vi "子VI-查看某框-只读穿透图模式.vi"(0 "输入框号（默认值0为整张图）":dbl format="%#_13g", 1 "框组":T3(array[cluster]), 3 "临界Z值":i32, 4 "弥散类缺陷灰度阈值":dbl caption="值", 5 "临界面积百分比值":dbl, 6 "分层缺陷的面积阈值":i32, 7 "预先配置的灰度阈值":dbl, 8 "穿透图原始路径":path, 9 "部位信息":string[](array[string])=["", "34.500000", "32.500000", "1121", "34", "54.955926", "分层类", "不合格", ""], 16 "产品规格":cluster{"产品长度（周长）（mm）":dbl, "产品宽度（母线长）（mm）":dbl}) -> (27 "全部检测结果":string[][](table))   [LabVIEW 2018]
uses:
  <vilib>/vision/NI_Vision_Development_Module.lvlib
panel:
  out "分层类缺陷低于阈值的累计面积":dbl
  out "中心Y":dbl
  out "中心X":dbl
  in  "格式字符串 4":string="%f"
  in  "分隔符（'\\'代码显示） 3":string="\t"
  out "?":string[][](table)
  in  "返回主界面":bool caption="辅助定性分析"
  in  "Tab Control":T1
  out "?":T2(plugin-control)
  out "Threshold Image":T2(plugin-control)
  out "Threshold Image":T2(plugin-control)
  in  "格式字符串 3":string="%f"
  in  "分隔符（'\\'代码显示） 2":string="\t"
  out "弥散缺陷个数":i32
  out "分层缺陷个数":i32
  out "合格？ 弥散类":string="fencengThreshold"
  out "合格？分层类":string="fencengThreshold"
  out "弥散测量结果":dbl[][](array[numeric])
  out "弥散类检测结果":string[][](table)
  out "?":string
  out "面积 (pixels)":i32
  in  "格式字符串 2":string="%f"
  in  "分隔符（'\\'代码显示）":string="\t"
  out "分层测量结果":dbl[][](array[numeric])
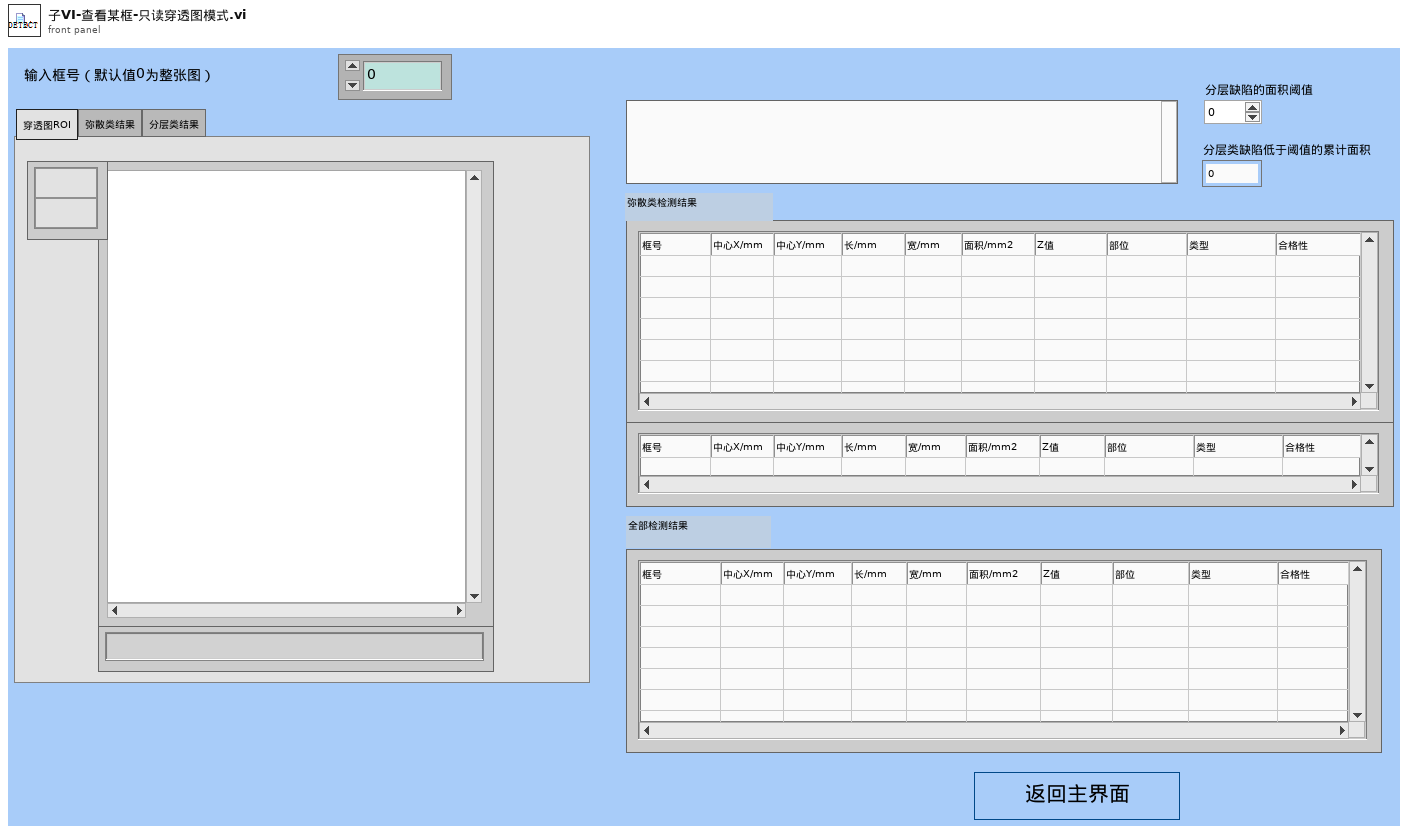
[diagram p1: front panel]
types:
  T1 = typedef "控件2.ctl" = enum32{"穿透图ROI", "弥散类结果", "分层类结果"}
  T2 = typedef "IMAQ Image.ctl" = refnum<image>
  T3 = cluster{"Global Rectangle":i32[], "Contours":cluster{"Contour Type":u32, "ROI Type":u32, "Points":i32[]}[]}[]
  T4 = cluster{"Zoom Tool":bool, "Selection Tool":bool, "Pan Tool":bool, "Point Tool":bool, "Line Tool":bool, "Rectangle Tool":bool, "Rotated Rectangle Tool":bool, "Polyline Tool":bool, "Polygon Tool":bool, "Freehand Tool":bool, "Closed Freehand Tool":bool, "Ellipse Tool":bool, "Annulus Tool":bool}
  T5 = typedef "Image Type" = u32
  T6 = cluster{"Global Rectangle":i32[], "Contours":cluster{"Contour Type":u32, "ROI Type":u32, "Points":i32[]}[]}
  T7 = cluster{"histogram":u32[], "Minimal Value":sgl, "Maximal Value":sgl, "Starting Value":sgl, "Interval Width":sgl, "Mean Value":sgl, "Standard  Variation":sgl, "Area (pixels)":i32}
  T8 = cluster{"Area":dbl, "Number of Holes":dbl, "Bounding Rect":cluster{"Left":dbl, "Top":dbl, "Right":dbl, "Bottom":dbl}, "Center of Mass":cluster{"X":dbl, "Y":dbl}, "Orientation":dbl, "Dimensions":cluster{"Width":dbl, "Height":dbl}}[]
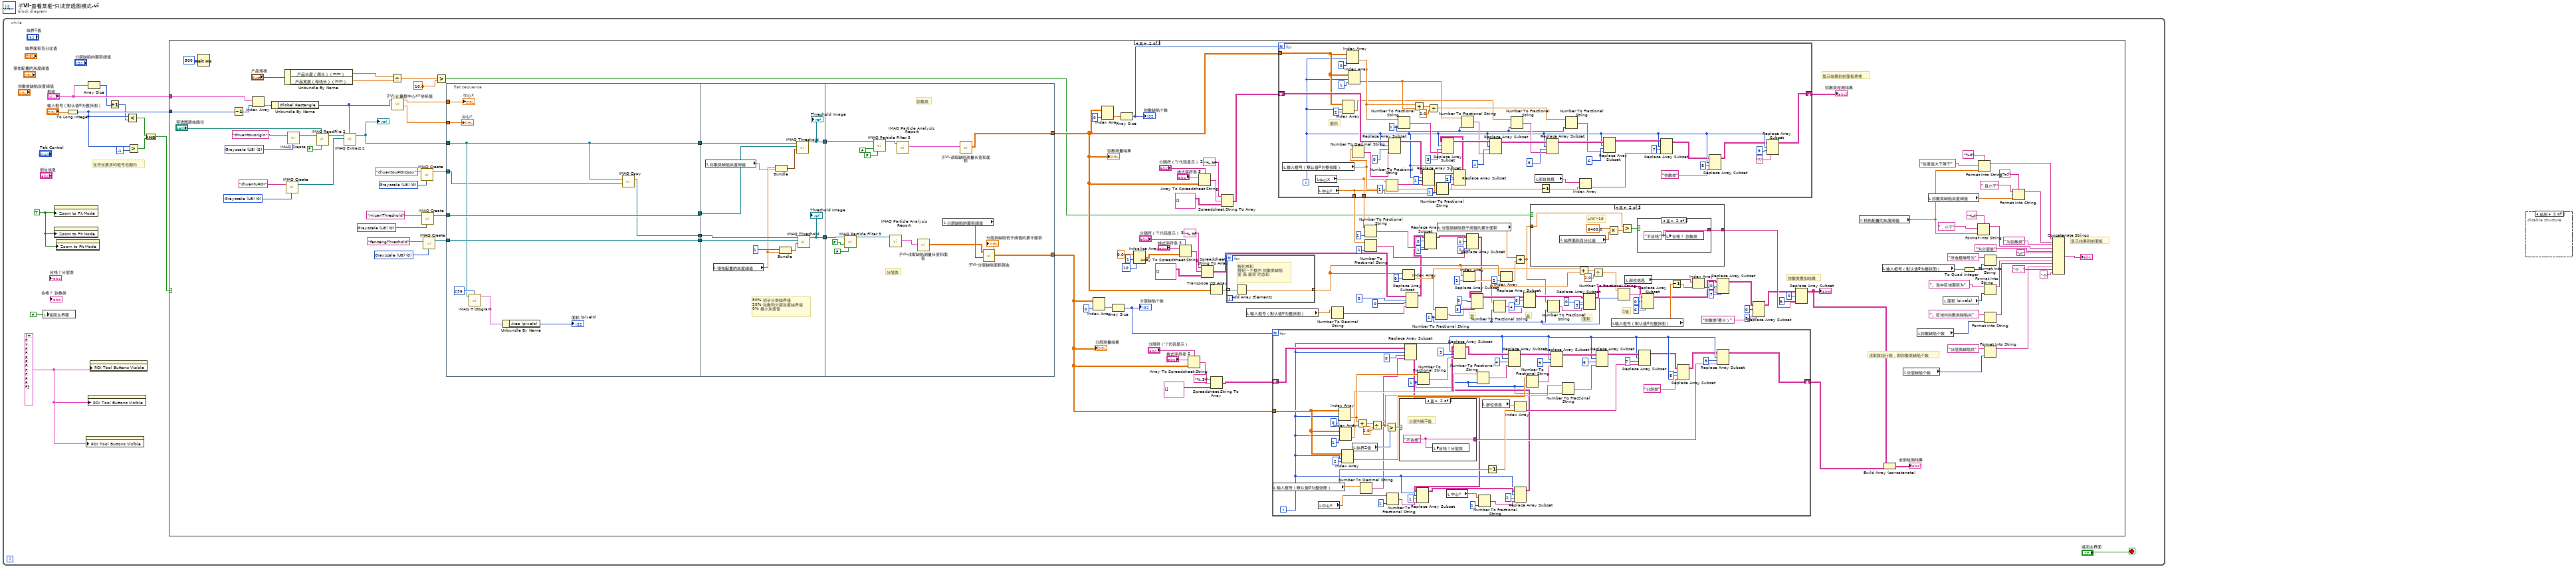
[diagram p0: block diagram]
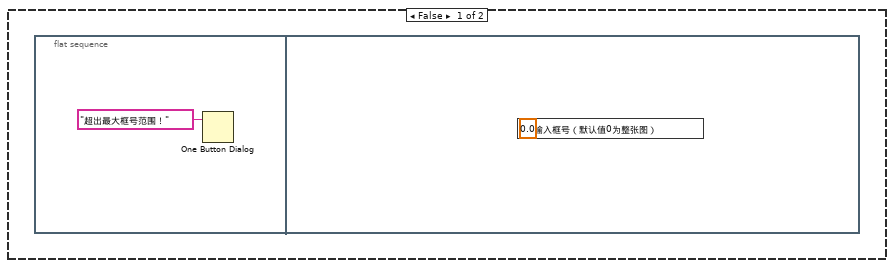
[diagram p2: hidden frame]
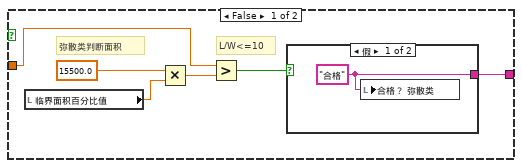
[diagram p3: hidden frame]
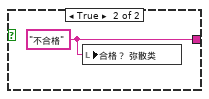
[diagram p4: hidden frame]
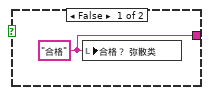
[diagram p5: hidden frame]
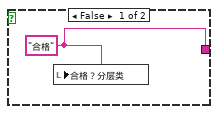
[diagram p6: hidden frame]
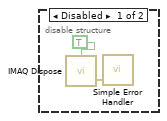
[diagram p7: hidden frame]
diagram:
  n1 = while {
    stop <- "返回主界面" stop-if-true
    w3 = T4 {"Zoom Tool"=TRUE, "Selection Tool"=FALSE, "Pan Tool"=TRUE, "Point Tool"=FALSE, "Line Tool"=FALSE, "Rectangle Tool"=FALSE, "Rotated Rectangle Tool"=FALSE, "Polyline Tool"=FALSE, "Polygon Tool"=FALSE, "Freehand Tool"=FALSE, "Closed Freehand Tool"=FALSE, "Ellipse Tool"=FALSE, "Annulus Tool"=FALSE} ("ROI Tool Buttons Visible:All Elements")
    w11 = TRUE ("Zoom to Fit Mode")
    # "在符合要求的框号范围内"
    n2 = local write "返回主界面"(FALSE ("stop")) -> ()
    n3 = property class="ImageControl"("Zoom to Fit Mode"=w11) -> ()  [unwired: 2 in, 2 out]
    n4 = property class="ImageControl"("Zoom to Fit Mode"=w11) -> ()  [unwired: 2 in, 2 out]
    n5 = property class="ImageControl"("Zoom to Fit Mode"=w11) -> ()  [unwired: 2 in, 2 out]
    n6 = To Long Integer(number="输入框号（默认值0为整张图）") -> (32bit integer=w5:i32)
    n7 = property class="ImageControl"("ROI Tool Buttons Visible"=w3) -> ()  [unwired: 2 in, 2 out]
    n8 = Array Size(array="框组") -> (size(s)=w2:i32)
    n9 = property class="ImageControl"("ROI Tool Buttons Visible"=w3) -> ()  [unwired: 2 in, 2 out]
    n10 = property class="ImageControl"("ROI Tool Buttons Visible"=w3) -> ()  [unwired: 2 in, 2 out]
    n11 = Increment(x=w2) -> (x+1=w1:i32)
    n12 = Less?(x=w5, y=w1) -> (x < y?=w7:bool)
    n13 = Greater?(x=w5, y=-1) -> (0:w6:bool)
    n14 = And(x=w7, y=w6) -> (x .and. y?=w8:bool)
    n15 = case shown="真" w8 {
      tunnel: "框组" -> [_ w106]
      tunnel: w5 -> [_ w105]
      frame False {
        n16 = flat-sequence {
          frame #0 {
            n17 = One Button Dialog(message="超出最大框号范围！" ("消息")) -> ()  [unwired: 1 in, 1 out]
          }
          frame #1 {
            n18 = local write "输入框号（默认值0为整张图）"(0.0 ("框号")) -> ()
          }
        }
      }
      frame True {
        w32 = i16 1 ("精度(6)")
        w131 = T5 0 items=["Grayscale (U8)", "Grayscale (I16)", "Grayscale (SGL)", "Complex (CSG)", "RGB (U32)", "HSL (U32)", "RGB (U64)", "Grayscale (U16)"] ("Image Type")
        w153 = T5 0 items=["Grayscale (U8)", "Grayscale (I16)", "Grayscale (SGL)", "Complex (CSG)", "RGB (U32)", "HSL (U32)", "RGB (U64)", "Grayscale (U16)"] ("Image Type")
        w154 = T5 0 items=["Grayscale (U8)", "Grayscale (I16)", "Grayscale (SGL)", "Complex (CSG)", "RGB (U32)", "HSL (U32)", "RGB (U64)", "Grayscale (U16)"] ("Image Type")
        w157 = T5 0 items=["Grayscale (U8)", "Grayscale (I16)", "Grayscale (SGL)", "Complex (CSG)", "RGB (U32)", "HSL (U32)", "RGB (U64)", "Grayscale (U16)"] ("Image Type")
        w170 = T5 0 items=["Grayscale (U8)", "Grayscale (I16)", "Grayscale (SGL)", "Complex (CSG)", "RGB (U32)", "HSL (U32)", "RGB (U64)", "Grayscale (U16)"] ("Image Type")
        # "Z值"
        # "面积"
        # "高"
        # "宽"
        # "弥散类累加结果"
        # "显示结果到前面板"
        # "读取数组行数，即弥散类缺陷个数"
        # "显示结果到前面板表格"
        n19 = Wait (ms)(milliseconds to wait=u32 500 ("等待时间（毫秒）")) -> ()  [unwired: 1 out]
        n20 = Decrement(x=w105) -> (x-1=w172:i32)
        n21 = Index Array(array=w106, index=w172) -> (element=w173:T6)
        n22 = Unbundle By Name(w173) -> ("Global Rectangle"=w48:i32[])
        n23 = Unbundle By Name("产品规格") -> ("产品长度（周长）（mm）"=w164:dbl, "产品宽度（母线长）（mm）"=w163:dbl)
        n24 = call "IMAQ Create"("Image Name"="chuantuROI", "Image Type"=w157) -> ("New Image"=w156:T2)  [unwired: 3 in, 1 out]
        n25 = call "IMAQ Create"("Image Name"="chuantouorigin", "Image Type"=w170) -> ("New Image"=w159:T2)  [unwired: 3 in, 1 out]
        n26 = call "IMAQ ReadFile 2"("Use File Path Image Type"=FALSE, "File Path"="穿透图原始路径", "Image"=w159) -> ("Image Out"=w160:T2)  [unwired: 4 in, 4 out]
        n27 = call "IMAQ Extract 2"("Optional Rectangle"=w48, "Image Dst"=w156, "Image Src"=w160) -> ("Image Dst Out"=w134:T2)  [unwired: 7 in, 1 out]
        "?" <- w134
        n28 = Divide(x=w164, y=w163) -> (x/y=w167:dbl)
        n29 = call "子VI-计算框中心XY坐标值.vi"("Global Rectangle"=w48) -> ("中心Y"=w28:dbl, "中心X"=w27:dbl)  [unwired: 9 in]
        n30 = call "IMAQ Create"("Image Name"="chuantouROIcopy", "Image Type"=w131) -> ("New Image"=w133:T2)  [unwired: 3 in, 1 out]
        n31 = call "IMAQ Create"("Image Name"="misanThreshold", "Image Type"=w153) -> ("New Image"=w148:T2)  [unwired: 3 in, 1 out]
        n32 = call "IMAQ Create"("Image Name"="fencengThreshold", "Image Type"=w154) -> ("New Image"=w147:T2)  [unwired: 3 in, 1 out]
        n33 = Greater?(x=w167, y=10.0) -> (0:w58:bool)
        n34 = flat-sequence {
          tunnel: [w261] -> w179
          tunnel: [w260] -> w178
          tunnel: [w256] -> w177
          tunnel: [w255] -> w176
          tunnel: w148 -> [w261]
          tunnel: w147 -> [w260]
          tunnel: w134 -> [w256]
          tunnel: w133 -> [w254]
          tunnel: w28 -> [w253]
          tunnel: w27 -> [w252]
          tunnel: w179 -> [w272]
          tunnel: w178 -> [w271]
          tunnel: [w267] -> w175
          tunnel: [w269] -> w174
          tunnel: w177 -> [w270]
          tunnel: w176 -> [w268]
          tunnel: [w277] -> w101
          tunnel: w175 -> [w283]
          tunnel: w174 -> [w282]
          tunnel: [w273] -> w16
          frame #0 {
            n35 = call "IMAQ Histogram"("Number of Classes"=256, "Image"=w256) -> ("Histogram Report"=w258:T7)  [unwired: 8 in, 1 out]
            n36 = Unbundle By Name(w258) -> ("Area (pixels)"=→"面积 (pixels)":i32)
            n37 = call "IMAQ Copy"("Image Dst"=w254, "Image Src"=w256) -> ("Image Dst Out"=w255:T2)  [unwired: 4 in, 1 out]
            "中心Y" <- w253
            "中心X" <- w252
          }
          frame #1 {
            # "50% 初步分类临界值\n20% 弥散和分层灰度临界值\n0% 最小灰度值"
            n38 = local read "弥散类缺陷灰度阈值"() -> (w262:dbl)
            n39 = local read "预先配置的灰度阈值"() -> (w263:dbl)
            n40 = Bundle("预先配置的灰度阈值"=w263, "弥散类缺陷灰度阈值"=w262) -> (w266:cluster{"预先配置的灰度阈值":dbl, "弥散类缺陷灰度阈值":dbl})  [unwired: 1 in]
            n41 = Bundle(1, "预先配置的灰度阈值"=w263) -> (w265:cluster{i32, "预先配置的灰度阈值":dbl})  [unwired: 1 in]
            n42 = call "IMAQ Threshold"("Range"=w266, "Image Dst"=w272, "Image Src"=w270) -> ("Image Dst Out"=w269:T2)  [unwired: 3 in, 5 out]
            "Threshold Image" <- w269
            n43 = call "IMAQ Threshold"("Range"=w265, "Image Dst"=w271, "Image Src"=w268) -> ("Image Dst Out"=w267:T2)  [unwired: 3 in, 5 out]
            "Threshold Image" <- w267
          }
          frame #2 {
            # "分层类"
            # "弥散类"
            n44 = call "IMAQ Particle Filter 3"("Image Src"=w283, "Keep/Remove Particles (F)"=FALSE, "Reject Border? (F)"=FALSE) -> ("Image Dst Out"=w281:T2)  [unwired: 10 in, 2 out]
            n45 = call "IMAQ Particle Filter 3"("Image Src"=w282, "Keep/Remove Particles (F)"=FALSE, "Reject Border? (F)"=FALSE) -> ("Image Dst Out"=w279:T2)  [unwired: 10 in, 2 out]
            n46 = call "IMAQ Particle Analysis Report"("Image"=w281) -> ("Particle Reports (Pixels)"=w280:T8)  [unwired: 5 in, 5 out]
            n47 = call "IMAQ Particle Analysis Report"("Image"=w279) -> ("Particle Reports (Pixels)"=w278:T8)  [unwired: 5 in, 5 out]
            n48 = call "子VI-读取缺陷测量长宽和面积.vi"("Particle Reports (Pixels)"=w280) -> ("测量结果"=w274:dbl[][])  [unwired: 10 in]
            n49 = local read "分层缺陷的面积阈值"() -> (w275:i32)
            n50 = call "子VI-读取缺陷测量长宽和面积.vi"("Particle Reports (Pixels)"=w278) -> ("测量结果"=w277:dbl[][])  [unwired: 10 in]
            n51 = call "子VI-分层缺陷面积筛选.vi"("计入分层缺陷的面积阈值"=w275, "分层测量结果"=w274) -> ("初始化的数组"=w273:dbl[][], "去掉的面积累计"=→"分层类缺陷低于阈值的累计面积":dbl)  [unwired: 8 in]
          }
        }
        n52 = Index Array(array=w16, index (col)=0 ("禁用的索引 (列)")) -> (element=w152:dbl[])  [unwired: 1 in]
        n53 = Index Array(array=w101, index (col)=0 ("禁用的索引 (列)")) -> (element=w150:dbl[])  [unwired: 1 in]
        n54 = Array Size(array=w152) -> (size(s)=w146:i32)
        "分层缺陷个数" <- w146
        n55 = Array Size(array=w150) -> (size(s)=w162:i32)
        "弥散缺陷个数" <- w162
        n56 = Initialize Array(0.0 ("元素"), 1 ("维数大小"), 10 ("维数大小")) -> (w89:dbl[][])
        n57 = Array To Spreadsheet String(delimiter (Tab)="分隔符（'\\'代码显示） 3", array=w89, 3:"格式字符串 4") -> (spreadsheet string=w92:string)
        n58 = Array To Spreadsheet String(delimiter (Tab)="分隔符（'\\'代码显示）", array=w16, 3:"格式字符串 2") -> (spreadsheet string=w143:string)
        n59 = Array To Spreadsheet String(delimiter (Tab)="分隔符（'\\'代码显示） 2", array=w101, 3:"格式字符串 3") -> (spreadsheet string=w138:string)
        n60 = Spreadsheet String To Array(format string="%.3f", spreadsheet string=w92, array type (2D Dbl)=string[][] [] ("Array")) -> (array=w88:string[][])  [unwired: 1 in]
        n61 = Transpose 2D Array(2D array=w101) -> (transposed array=w102:dbl[][])
        n62 = Spreadsheet String To Array(format string="%.3f" ("格式字符串"), spreadsheet string=w143, array type (2D Dbl)=string[][] [] ("Array")) -> (array=w141:string[][])  [unwired: 1 in]
        n63 = Spreadsheet String To Array(format string="%.3f", spreadsheet string=w138, array type (2D Dbl)=string[][] [] ("Array")) -> (array=w100:string[][])  [unwired: 1 in]
        n64 = for {
          tunnel: w102 -> [w197] mode=indexing
          tunnel: [w196] -> w75 mode=indexing
          # "按列求和 \n得到一个框内 弥散类缺陷\n宽 高 面积 的总和"
          n65 = Add Array Elements(numeric array=w197) -> (sum=w196:dbl)
        }
        n66 = local read "输入框号（默认值0为整张图）"() -> (w52:dbl)
        n67 = for {
          N: w146 -> [_]
          tunnel: w16 -> [w217]
          shift-right: [w225] -> w50
          shift-left: w141 -> [w233]
          i -> [w205]
          w198 = i16 1 ("精度(6)")
          n68 = local read "输入框号（默认值0为整张图）"() -> (w240:dbl)
          n69 = local read "中心X"() -> (w213:dbl)
          n70 = Index Array(array=w217, index (row)=w205, index (col)=0 ("禁用的索引 (列)")) -> (element=w224:dbl)
          n71 = Index Array(array=w217, index (row)=w205, index (col)=1 ("禁用的索引 (列)")) -> (element=w223:dbl)
          n72 = Index Array(array=w217, index (row)=w205, index (col)=2 ("索引 (列)")) -> (element=w216:dbl)
          n73 = local read "临界Z值"() -> (w247:i32)
          n74 = Add(x=w224, y=w223) -> (x+y=w248:dbl)
          n75 = Number To Decimal String(number=w240) -> (decimal integer string=w215:string)  [unwired: 1 in]
          n76 = Divide(x=w248, y=2.0) -> (x/y=w221:dbl)
          n77 = Greater?(x=w221, y=w247) -> (0:w249:bool)
          n78 = Number To Fractional String(number=w213, precision (6)=i16 1 ("精度(6)")) -> (F-format string=w208:string)  [unwired: 2 in]
          n79 = case shown="真" w249 {
            tunnel: [w250 w251] -> w219
            frame False {
              w250 = "合格" ("合格？")
              n80 = local write "合格？分层类"(w250) -> ()
            }
            frame True {
              w251 = "不合格" ("合格？")
              # "分层判断Z值"
              n81 = local write "合格？分层类"(w251) -> ()
            }
          }
          n82 = Replace Array Subset(array=w233, new element=w215, index (row)=w205, index (col)=0 ("索引 (列)")) -> (w212:string[][])
          n83 = Replace Array Subset(array=w212, new element=w208, index (row)=w205, index (col)=1 ("禁用的索引 (列)")) -> (w209:string[][])
          n84 = Number To Fractional String(number=w224, precision (6)=w198) -> (F-format string=w232:string)  [unwired: 2 in]
          n85 = local read "中心Y"() -> (w202:dbl)
          n86 = Number To Fractional String(number=w223, precision (6)=w198) -> (F-format string=w231:string)  [unwired: 2 in]
          n87 = Number To Fractional String(number=w202, precision (6)=i16 1 ("精度(6)")) -> (F-format string=w201:string)  [unwired: 2 in]
          n88 = local read "部位信息"() -> (w243:string[])
          n89 = Decrement(x=w240) -> (x-1=w242:dbl)
          n90 = Index Array(array=w243, index=w242) -> (element=w220:string)
          n91 = Replace Array Subset(array=w209, new element=w201, index (row)=w205, index (col)=2 ("索引 (列)")) -> (w207:string[][])
          n92 = Replace Array Subset(array=w207, new element=w232, index (row)=w205, index (col)=3 ("索引 (列)")) -> (w230:string[][])
          n93 = Replace Array Subset(array=w230, new element=w231, index (row)=w205, index (col)=4 ("索引 (列)")) -> (w229:string[][])
          n94 = Number To Fractional String(number=w216, precision (6)=w198) -> (F-format string=w228:string)  [unwired: 2 in]
          n95 = Replace Array Subset(array=w229, new element=w228, index (row)=w205, index (col)=5 ("索引 (列)")) -> (w227:string[][])
          n96 = Number To Fractional String(number=w221, precision (6)=w198) -> (F-format string=w222:string)  [unwired: 2 in]
          n97 = Replace Array Subset(array=w227, new element=w222, index (row)=w205, index (col)=6 ("索引 (列)")) -> (w226:string[][])
          n98 = Replace Array Subset(array=w226, new element=w220, index (row)=w205, index (col)=7 ("索引 (列)")) -> (w204:string[][])
          n99 = Replace Array Subset(array=w204, new element="分层类" ("新元素/子数组"), index (row)=w205, index (col)=8 ("索引 (列)")) -> (w203:string[][])
          n100 = Replace Array Subset(array=w203, new element=w219, index (row)=w205, index (col)=9 ("索引 (列)")) -> (w225:string[][])
        }
        n101 = for {
          N: w162 -> [_]
          tunnel: w101 -> [w308]
          shift-right: [w323] -> w135
          shift-left: w100 -> [w328]
          tunnel: [w289] -> w26
          tunnel: [w288] -> w25
          i -> [w296]
          w292 = i16 1 ("精度(6)")
          # "面积"
          n102 = local read "输入框号（默认值0为整张图）"() -> (w311:dbl)
          n103 = local read "中心X"() -> (w289:dbl)
          n104 = local read "中心Y"() -> (w288:dbl)
          n105 = Index Array(array=w308, index (row)=w296, index (col)=2 ("索引 (列)")) -> (element=w307:dbl)
          n106 = Index Array(array=w308, index (row)=w296, index (col)=0 ("禁用的索引 (列)")) -> (element=w317:dbl)
          n107 = Index Array(array=w308, index (row)=w296, index (col)=1 ("禁用的索引 (列)")) -> (element=w316:dbl)
          n108 = Number To Decimal String(number=w311) -> (decimal integer string=w305:string)  [unwired: 1 in]
          n109 = Number To Fractional String(number=w289, precision (6)=i16 1 ("精度(6)")) -> (F-format string=w301:string)  [unwired: 2 in]
          n110 = Replace Array Subset(array=w328, new element=w305, index (row)=w296, index (col)=0 ("索引 (列)")) -> (w304:string[][])
          n111 = Number To Fractional String(number=w317, precision (6)=w292) -> (F-format string=w322:string)  [unwired: 2 in]
          n112 = Add(x=w317, y=w316) -> (x+y=w319:dbl)
          n113 = Replace Array Subset(array=w304, new element=w301, index (row)=w296, index (col)=1 ("禁用的索引 (列)")) -> (w303:string[][])
          n114 = Divide(x=w319, y=2.0) -> (x/y=w315:dbl)
          n115 = Number To Fractional String(number=w288, precision (6)=i16 1 ("精度(6)")) -> (F-format string=w299:string)  [unwired: 2 in]
          n116 = Replace Array Subset(array=w303, new element=w299, index (row)=w296, index (col)=2 ("禁用的索引 (列)")) -> (w302:string[][])
          n117 = Replace Array Subset(array=w302, new element=w322, index (row)=w296, index (col)=3 ("索引 (列)")) -> (w327:string[][])
          n118 = Number To Fractional String(number=w316, precision (6)=w292) -> (F-format string=w321:string)  [unwired: 2 in]
          n119 = Replace Array Subset(array=w327, new element=w321, index (row)=w296, index (col)=4 ("索引 (列)")) -> (w326:string[][])
          n120 = Number To Fractional String(number=w307, precision (6)=w292) -> (F-format string=w320:string)  [unwired: 2 in]
          n121 = local read "部位信息"() -> (w313:string[])
          n122 = Decrement(x=w311) -> (x-1=w312:dbl)
          n123 = Replace Array Subset(array=w326, new element=w320, index (row)=w296, index (col)=5 ("索引 (列)")) -> (w325:string[][])
          n124 = Number To Fractional String(number=w315, precision (6)=w292) -> (F-format string=w314:string)  [unwired: 2 in]
          n125 = Index Array(array=w313, index=w312) -> (element=w310:string)
          n126 = Replace Array Subset(array=w325, new element=w314, index (row)=w296, index (col)=6 ("索引 (列)")) -> (w324:string[][])
          n127 = Replace Array Subset(array=w324, new element=w310, index (row)=w296, index (col)=7 ("索引 (列)")) -> (w294:string[][])
          n128 = Replace Array Subset(array=w294, new element="弥散类" ("新元素/子数组"), index (row)=w296, index (col)=8 ("索引 (列)")) -> (w293:string[][])
          n129 = Replace Array Subset(array=w293, new element="\\" ("新元素/子数组"), index (row)=w296, index (col)=9 ("索引 (列)")) -> (w323:string[][])
        }
        "弥散类检测结果" <- w135
        n130 = Number To Decimal String(number=w52) -> (decimal integer string=w47:string)  [unwired: 1 in]
        n131 = Number To Fractional String(number=w26, precision (6)=i16 1 ("精度(6)")) -> (F-format string=w41:string)  [unwired: 2 in]
        n132 = Number To Fractional String(number=w25, precision (6)=i16 1 ("精度(6)")) -> (F-format string=w33:string)  [unwired: 2 in]
        n133 = Index Array(array=w75, index=0 ("索引")) -> (element=w54:dbl)
        n134 = Replace Array Subset(array=w88, new element=w47, index (row)=0 ("禁用的索引 (行)"), index (col)=0 ("索引 (列)")) -> (w36:string[][])
        n135 = Replace Array Subset(array=w36, new element=w41, index (row)=0 ("索引 (行)"), index (col)=1 ("索引 (列)")) -> (w35:string[][])
        n136 = Number To Fractional String(number=w54, precision (6)=w32) -> (F-format string=w84:string)  [unwired: 2 in]
        n137 = local read "分层类缺陷低于阈值的累计面积"() -> (w19:dbl)
        n138 = Index Array(array=w75, index=1 ("索引")) -> (element=w53:dbl)
        n139 = Replace Array Subset(array=w35, new element=w33, index (row)=0 ("索引 (行)"), index (col)=2 ("索引 (列)")) -> (w34:string[][])
        n140 = Replace Array Subset(array=w34, new element=w84, index (row)=0 ("索引 (行)"), index (col)=3 ("索引 (列)")) -> (w82:string[][])
        n141 = Number To Fractional String(number=w53, precision (6)=w32) -> (F-format string=w74:string)  [unwired: 2 in]
        n142 = Index Array(array=w75, index=2 ("索引")) -> (element=w18:dbl)
        n143 = Add(x=w19, y=w18) -> (x+y=w17:dbl)
        n144 = Replace Array Subset(array=w82, new element=w74, index (row)=0 ("索引 (行)"), index (col)=4 ("禁用的索引 (列)")) -> (w77:string[][])
        n145 = case shown="真" w58 {
          tunnel: [w184 w192] -> w55
          tunnel: w17 -> [w180 w188]
          frame False {
            # "弥散类判断面积"
            # "L/W<=10"
            n146 = local read "临界面积百分比值"() -> (w182:dbl)
            n147 = Multiply(x=15500.0, y=w182) -> (x*y=w181:dbl)
            n148 = Greater?(x=w180, y=w181) -> (0:w185:bool)
            n149 = case shown="假" w185 {
              tunnel: [w186 w187] -> w184
              frame False {
                w186 = "合格" ("合格？")
                n150 = local write "合格？ 弥散类"(w186) -> ()
              }
              frame True {
                w187 = "不合格" ("合格？")
                n151 = local write "合格？ 弥散类"(w187) -> ()
              }
            }
          }
          frame True {
            # "L/W>10"
            n152 = local read "临界面积百分比值"() -> (w189:dbl)
            n153 = Multiply(x=6400.0, y=w189) -> (x*y=w191:dbl)
            n154 = Greater?(x=w188, y=w191) -> (0:w193:bool)
            n155 = case shown="真" w193 {
              tunnel: [w194 w195] -> w192
              frame False {
                w194 = "合格" ("合格？")
                n156 = local write "合格？ 弥散类"(w194) -> ()
              }
              frame True {
                w195 = "不合格" ("合格？")
                n157 = local write "合格？ 弥散类"(w195) -> ()
              }
            }
          }
        }
        n158 = Number To Fractional String(number=w17, precision (6)=w32) -> (F-format string=w73:string)  [unwired: 2 in]
        n159 = Add(x=w54, y=w53) -> (x+y=w72:dbl)
        n160 = Replace Array Subset(array=w77, new element=w73, index (row)=0 ("索引 (行)"), index (col)=5 ("索引 (列)")) -> (w66:string[][])
        n161 = Divide(x=w72, y=2.0) -> (x/y=w70:dbl)
        n162 = local read "输入框号（默认值0为整张图）"() -> (w65:dbl)
        n163 = Number To Fractional String(number=w70, precision (6)=w32) -> (F-format string=w69:string)  [unwired: 2 in]
        n164 = local read "部位信息"() -> (w63:string[])
        n165 = Replace Array Subset(array=w66, new element=w69, index (row)=0 ("索引 (行)"), index (col)=6 ("索引 (列)")) -> (w59:string[][])
        n166 = Decrement(x=w65) -> (x-1=w64:dbl)
        n167 = Index Array(array=w63, index=w64) -> (element=w62:string)
        n168 = Replace Array Subset(array=w59, new element=w62, index (row)=0 ("索引 (行)"), index (col)=7 ("索引 (列)")) -> (w46:string[][])
        n169 = Replace Array Subset(array=w46, new element="弥散类(累计）" ("新元素/子数组"), index (row)=0 ("索引 (行)"), index (col)=8 ("禁用的索引 (列)")) -> (w45:string[][])
        n170 = Replace Array Subset(array=w45, new element=w55, index (row)=0 ("索引 (行)"), index (col)=9 ("索引 (列)")) -> (w51:string[][])
        "?" <- w51
        n171 = local read "预先配置的灰度阈值"() -> (w29:dbl)
        n172 = local read "输入框号（默认值0为整张图）"() -> (w123:dbl)
        n173 = Build Array (concatenate)(w51, w50) -> (→"全部检测结果":string[][])
        n174 = local read "分层缺陷个数"() -> (w108:i32)
        n175 = local read "弥散缺陷个数"() -> (w107:i32)
        n176 = local read "弥散类缺陷灰度阈值"() -> (w22:dbl)
        n177 = local read "面积 (pixels)"() -> (w126:i32)
        n178 = To Quad Integer(1:w123) -> (0:w124:i64)
        n179 = Format Into String(format string="%d" ("格式字符串"), initial string="，小于" ("初始字符串"), w29) -> (resulting string=w127:string)  [unwired: 1 in, 1 out]
        n180 = Format Into String(format string="%d" ("格式字符串"), initial string="灰度值大于等于" ("初始字符串"), w29) -> (resulting string=w20:string)  [unwired: 1 in, 1 out]
        n181 = Format Into String(initial string="所选框编号为" ("初始字符串"), w124) -> (resulting string=w122:string)  [unwired: 2 in, 1 out]
        n182 = Format Into String(initial string="。选中区域面积为" ("字符串"), w126) -> (resulting string=w128:string)  [unwired: 2 in, 1 out]
        n183 = Format Into String(initial string="。区域内弥散类缺陷共" ("初始字符串"), w107) -> (resulting string=w129:string)  [unwired: 2 in, 1 out]
        n184 = Format Into String(initial string="分层类缺陷共" ("初始字符串"), w108) -> (resulting string=w130:string)  [unwired: 2 in, 1 out]
        n185 = Format Into String(format string="%d" ("格式字符串"), initial string=" 且小于" ("初始字符串"), w22) -> (resulting string=w21:string)  [unwired: 1 in, 1 out]
        n186 = Concatenate Strings(w20, w21, "为弥散类" ("初始字符串"), w127, "为分层类" ("初始字符串"), "\n", w122, w128, w129, "个，" ("字符串"), w130, "个" ("字符串")) -> (→"?":string)
        "分层测量结果" <- w16
        "弥散测量结果" <- w101
      }
    }
  }
  n187 = disable-structure shown="启用" {
    frame Disabled {
      n188 = call "IMAQ Dispose"("All Images? (No)"=TRUE) -> ("error out"=w339:errorcluster)  [unwired: 5 in]
      n189 = call <vilib>:"Simple Error Handler.vi"("error in (no error)"=w339) -> ()  [unwired: 4 in, 5 out]
    }
    frame Enabled {
    }
  }
